vi "Zaber Expert - Simultaneous Requests.vi"() -> ()   [LabVIEW 2015]
doc: "This example sends the same requests to two devices simultaneously. It sends a request to each device, and then waits for two responses before sending the next pair of requests.\nThe block diagram demonstrates using multiple writes with blocking reads to send simultaneous requests to two devices, instead of waiting for the first device's command to complete before sending the second one."
uses:
  ZaberTSeries.lvlib
  Public/Utility/Response.ctl
panel:
  in  "Second Device Number":u8=2
  out "Responses":T1[](array[typedef]) {"Command" items=["Constant Speed Tracking"=8, "Echo"=55, "Error"=255, "Home"=1, "Limit Active"=9, "Manual Move Tracking"=10, "Move Absolute"=20, "Move at Constant Speed"=22, "Move Relative"=21, "Renumber"=2, "Restore Settings"=36, "Stop"=23]}
  in  "Move Size":i32=10000
  in  "Device Number":u8=1
  in  "Move Count":i32=5
  in  "VISA resource name":refnum<visa-resource-name>
  # "This sends the same requests to two devices simultaneously. It sends a request\nto each device, and then waits for two responses before sending the next pair\nof requests.\nType Ctrl-E to see how the block diagram is wired."
  # "Don't use device 0."
  # "Don't use device 0."
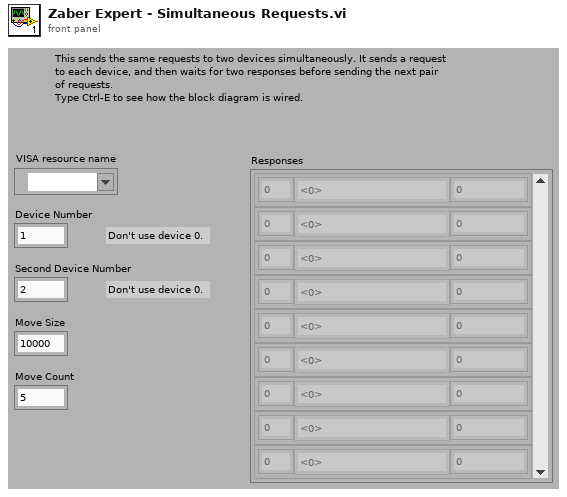
[diagram p1: front panel]
types:
  T1 = typedef "ZaberTSeries.lvlib/Response.ctl" = cluster{"Device Number":u8, "Command":u8, "Data":i32}
  T2 = cluster{"Device Number":u8, "Command":u8, "Data":i32, "Response Count":i32}
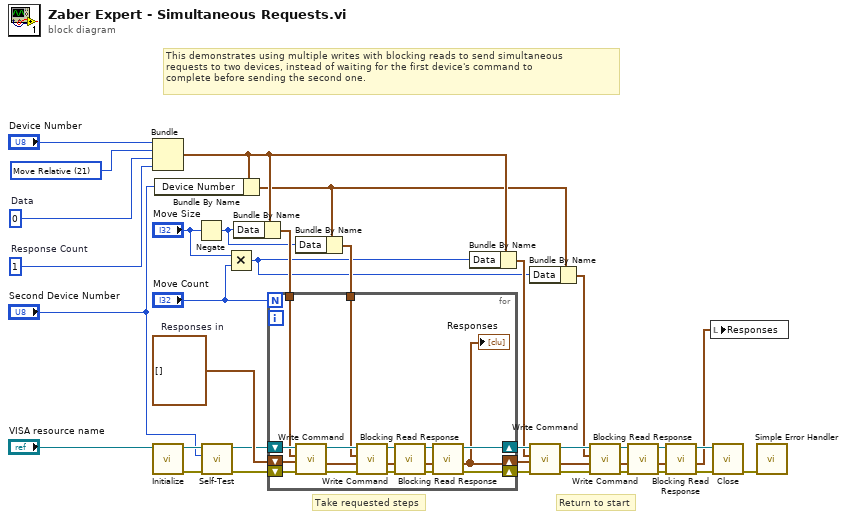
[diagram p0: block diagram]
diagram:
  w25 = 0  # Data
  w29 = 1  # Response Count
  w30 = u8 21 items=["Echo"=55, "Home"=1, "Move Absolute"=20, "Move Relative"=21, "Move at Constant Speed"=22, "Renumber"=2, "Restore Settings"=36, "Stop"=23] ("Command")
  w32 = T1[] []  # Responses in
  # "This demonstrates using multiple writes with blocking reads to send simultaneous\nrequests to two devices, instead of waiting for the first device's command to\ncomplete before sending the second one."
  # "Return to start"
  # "Take requested steps"
  n1 = Bundle("Device Number"="Device Number", "Command"=w30, "Data"=w25, "Response Count"=w29) -> (w23:T2)  [unwired: 1 in]
  n2 = call "Initialize.vi"("VISA resource name"="VISA resource name") -> ("error out"=w5:errorcluster, "VISA resource name out"=w4:refnum<visa-resource-name>)  [unwired: 8 in, 1 out]
  n3 = Bundle By Name(cluster=w23, "Device Number"="Second Device Number") -> (w17:T2)
  n4 = Negate(x="Move Size") -> (-x=w22:i32)
  n5 = call "Self-Test.vi"("error in (no error)"=w5, "Device Number"="Second Device Number", "VISA resource name"=w4) -> ("error out"=w3:errorcluster, "VISA resource name out"=w2:refnum<visa-resource-name>)  [unwired: 5 in, 2 out]
  n6 = Multiply(x="Move Size", y="Move Count") -> (x*y=w16:i32)
  n7 = Bundle By Name(cluster=w23, "Data"=w22) -> (w24:T2)
  n8 = Bundle By Name(cluster=w17, "Data"=w22) -> (w21:T2)
  n9 = for {
    N: "Move Count" -> [_]
    shift-right: [w39] -> w31
    shift-left: w32 -> [w52]
    shift-right: [w38] -> w34
    shift-left: w3 -> [w54]
    tunnel: w24 -> [w51]
    shift-right: [w42] -> w35
    shift-left: w2 -> [w53]
    tunnel: w21 -> [w47]
    n10 = call "Write Command.vi"("error in (no error)"=w54, "Responses in"=w52, "Request"=w51, "VISA resource name"=w53) -> ("error out"=w48:errorcluster, "Responses out"=w49:T1[], "VISA resource name out"=w50:refnum<visa-resource-name>)  [unwired: 5 in]
    n11 = call "Write Command.vi"("error in (no error)"=w48, "Responses in"=w49, "Request"=w47, "VISA resource name"=w50) -> ("error out"=w44:errorcluster, "Responses out"=w45:T1[], "VISA resource name out"=w46:refnum<visa-resource-name>)  [unwired: 5 in]
    n12 = call "Blocking Read Response.vi"("error in (no error)"=w44, "Responses in"=w45, "VISA resource name"=w46) -> ("error out"=w40:errorcluster, "Responses out"=w41:T1[], "VISA resource name out"=w43:refnum<visa-resource-name>)  [unwired: 5 in, 1 out]
    n13 = call "Blocking Read Response.vi"("error in (no error)"=w40, "Responses in"=w41, "VISA resource name"=w43) -> ("error out"=w38:errorcluster, "Responses out"=w39:T1[], "VISA resource name out"=w42:refnum<visa-resource-name>)  [unwired: 5 in, 1 out]
    "Responses" <- w39
  }
  n14 = Bundle By Name(cluster=w23, "Data"=w16) -> (w33:T2)
  n15 = Bundle By Name(cluster=w17, "Data"=w16) -> (w15:T2)
  n16 = call "Write Command.vi"("error in (no error)"=w34, "Responses in"=w31, "Request"=w33, "VISA resource name"=w35) -> ("error out"=w20:errorcluster, "Responses out"=w19:T1[], "VISA resource name out"=w18:refnum<visa-resource-name>)  [unwired: 5 in]
  n17 = call "Write Command.vi"("error in (no error)"=w20, "Responses in"=w19, "Request"=w15, "VISA resource name"=w18) -> ("error out"=w13:errorcluster, "Responses out"=w12:T1[], "VISA resource name out"=w14:refnum<visa-resource-name>)  [unwired: 5 in]
  n18 = call "Blocking Read Response.vi"("error in (no error)"=w13, "Responses in"=w12, "VISA resource name"=w14) -> ("error out"=w10:errorcluster, "Responses out"=w11:T1[], "VISA resource name out"=w9:refnum<visa-resource-name>)  [unwired: 5 in, 1 out]
  n19 = call "Blocking Read Response.vi"("error in (no error)"=w10, "Responses in"=w11, "VISA resource name"=w9) -> ("error out"=w6:errorcluster, "Responses out"=w7:T1[], "VISA resource name out"=w8:refnum<visa-resource-name>)  [unwired: 5 in, 1 out]
  n20 = local write "Responses"(w7) -> ()
  n21 = call "Close.vi"("error in (no error)"=w6, "VISA resource name"=w8) -> ("error out"=w37:errorcluster)  [unwired: 8 in, 1 out]
  n22 = call <vilib>:"Simple Error Handler.vi"("error in (no error)"=w37) -> ()  [unwired: 4 in, 5 out]
